vi "ParametersUpdate.vi"(8 "error in (no error)":errorcluster, 10 "Signal Parameters":T1 {"Amplitude" format="%#_2g V"; "Frequency" format="%d Hz"}, 11 "Signal Generation in":refnum<class "Signal Generation.lvclass">) -> (0 "error out":errorcluster, 3 "Signal Generation out":refnum<class "Signal Generation.lvclass">)   [LabVIEW 2020, in "Signal Generation.lvlib" / "Signal Generation.lvclass"]
uses:
  Signal Generation.lvclass
  Controls/SignalParamTD.ctl
  Controls/SignalShapeTD.ctl
  Signal Generation.lvclass/Signal Generation.ctl
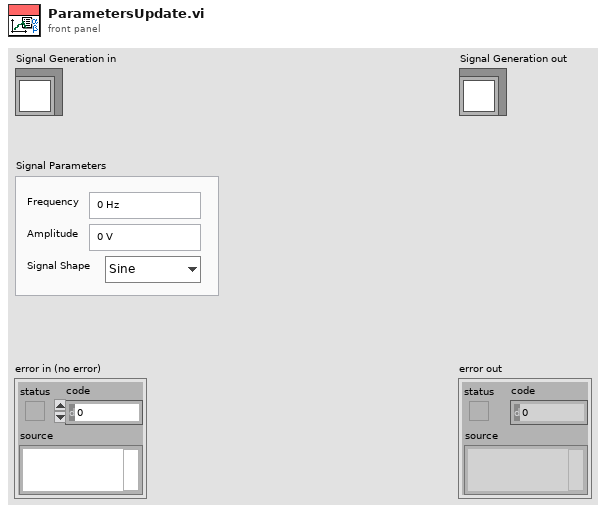
[diagram p1: front panel]
types:
  T1 = typedef "SignalParamTD.ctl" = cluster{"Frequency":u32, "Amplitude":dbl, "Signal Shape":T2}
  T2 = typedef "SignalShapeTD.ctl" = enum16{"Sine", "Square", "Triangle"}
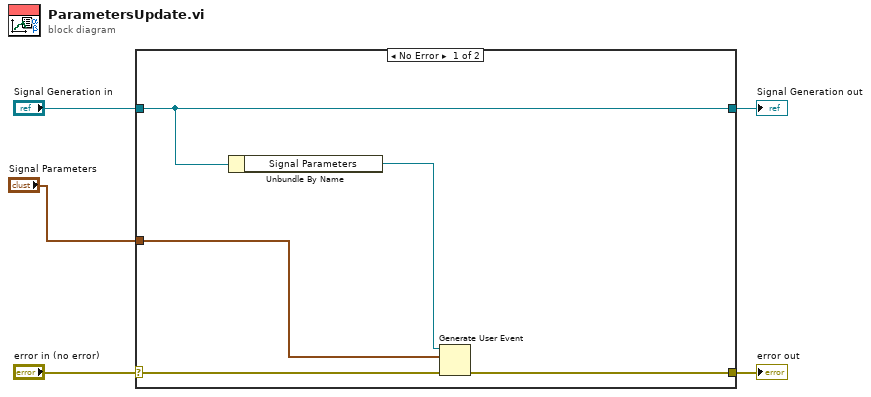
[diagram p0: block diagram]
diagram:
  n1 = case shown="No Error" "error in (no error)" {
    selector: "error in (no error)" -> [w9 w12]
    tunnel: [w8 w12] -> w4
    tunnel: [w10 w11] -> w2
    tunnel: "Signal Generation in" -> [w10 w11]
    tunnel: "Signal Parameters" -> [w6 _]
    frame No Error {
      n2 = Unbundle By Name(w10) -> ("Signal Parameters"=w7:refnum<user-event>)
      n3 = Generate User Event(user event=w7, event data cluster=w6, error in=w9) -> (error out=w8:errorcluster)  [unwired: 1 in, 1 out]
    }
    frame Error {
    }
  }
  "error out" <- w4
  "Signal Generation out" <- w2
